vi "X_2.84_SUBVI_LogWriter.vi"(9 "Gen goende array ind":string[](array[string]), 11 "Ny string":string) -> (2 "Gen goende aray out":string[](array[string]), 3 "Log out":string)   [LabVIEW 2022 SP3]
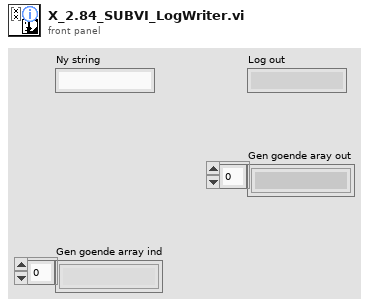
[diagram p1: front panel]
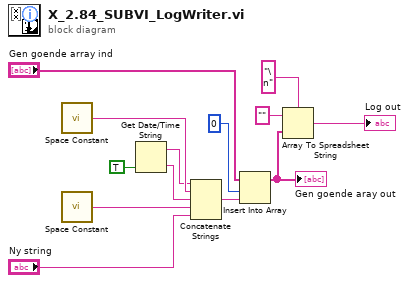
[diagram p0: block diagram]
diagram:
  n1 = call <vilib>:"Space Constant.vi"() -> ("String"=w9:string)
  n2 = call <vilib>:"Space Constant.vi"() -> ("String"=w11:string)
  n3 = Get Date/Time String(want seconds? (F)=TRUE) -> (date string=w8:string, time string=w10:string)  [unwired: 2 in]
  n4 = Concatenate Strings(w8, w9, w10, w11, "Ny string") -> (w13:string)
  n5 = Insert Into Array(array="Gen goende array ind", index=0 ("Log index"), new element=w13) -> (w5:string[])
  "Gen goende aray out" <- w5
  n6 = Array To Spreadsheet String(delimiter (Tab)="\n", array=w5, 3:"" ("format string")) -> (spreadsheet string=→"Log out":string)
